vi "CRYUpdate CDD Sub.vi"(10 "sData":string, 11 "sAction":string) -> (0 "Document Data Out":string, 2 "Flatten Data Out":string)   [LabVIEW 2013]
uses:
  CRYProject Editor Global.vi
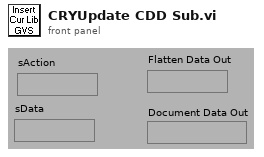
[diagram p1: front panel]
types:
  T1 = typedef "CRYTS.ctl" = cluster{"No.TS":u16, "TS File Path":path, "TS Name":string, "EditStepName":string, "Steps":T2[], "New State":bool, "Change State":bool, "Flattened CurveLib Data":string, "Document Data":string, "EditStepNo":u16, "Operator Start File":string, "Sequence Type":string, "Sequence Language":string}
  T2 = typedef "CRYStep.ctl" = cluster{"No.VI":i32, "Category":string, "StepName":string, "Seq setup flattened":string, "Comment":string, "Steps config.":bool[], "Jump config":i32[], "Start":dbl, "Increment":dbl, "Name":string, "Unit":string, "Y data":u16, "Y prefix":string, "Y dB ref":dbl, "Y unit":string, "Repeat State Array":cluster{"Start":dbl, "Increment":dbl, "Count":i32, "Num":i32}[]}
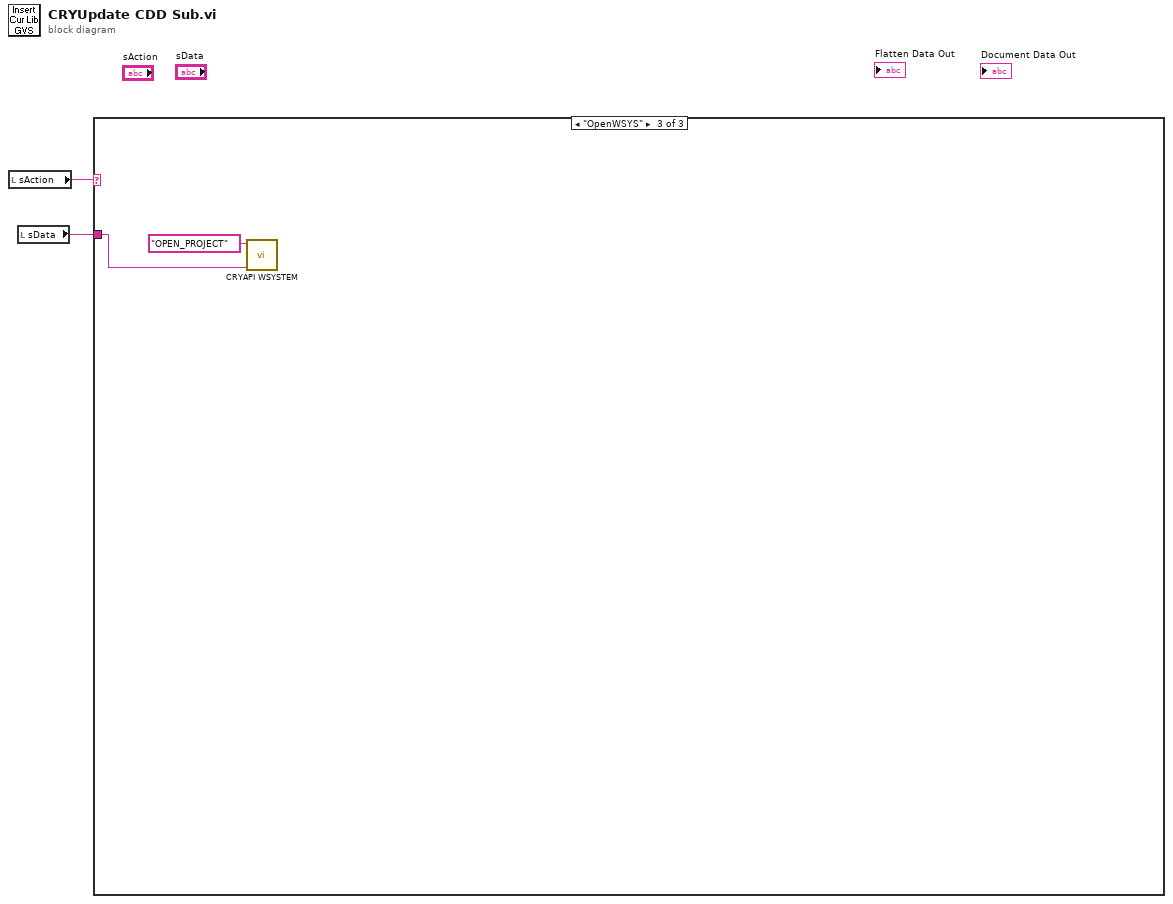
[diagram p0: block diagram]
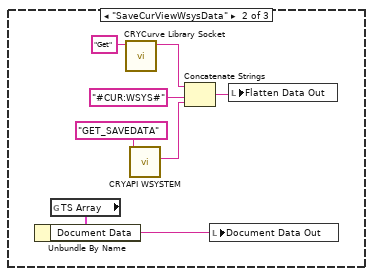
[diagram p3: hidden frame]
diagram:
  n1 = local read "sAction"() -> (w2:string)
  n2 = local read "sData"() -> (w1:string)
  n3 = case shown="\"OpenWSYS\"" w2 {
    tunnel: w1 -> [_ _ w12]
    frame Default {
    }
    frame "SaveCurViewWsysData" {
      n4 = global read "CRYProject Editor Global.vi" "TS Array"() -> (w4:T1)
      n5 = Unbundle By Name(w4) -> ("Document Data"=w3:string)
      n6 = call "CRYCurve Library Socket.vi"("sAction"="Get") -> ("sDataOut"=w5:string)  [unwired: 10 in]
      n7 = call "CRYAPI WSYSTEM.vi"("sAction"="GET_SAVEDATA") -> ("sData_Out"=w7:string)  [unwired: 7 in, 3 out]
      n8 = Concatenate Strings(w5, "#CUR:WSYS#", w7) -> (w9:string)
      n9 = local write "Document Data Out"(w3) -> ()
      n10 = local write "Flatten Data Out"(w9) -> ()
    }
    frame "OpenWSYS" {
      n11 = call "CRYAPI WSYSTEM.vi"("sData"=w12, "sAction"="OPEN_PROJECT") -> ()  [unwired: 6 in, 4 out]
    }
  }
